vi "getEffWave.vi"(8 "error in (no error)":errorcluster, 10 "Filter Type":T1, 11 "OptStateEsti in":refnum<class "OptStateEsti.lvclass">) -> (0 "error out":errorcluster, 2 "Effective Wavelength  (um)":dbl, 3 "OptStateEsti out":refnum<class "OptStateEsti.lvclass">)   [LabVIEW 2016, in "OptStateEsti.lvclass"]
doc: "Get the effective wavelength in um based on the active filter type (u, g, r, i, z, y, ref). It is noted that \"ref\" means the monochromatic reference wavelength."
uses:
  OptStateEsti.lvclass
  StrictDef/FilterType.ctl
  OptStateEsti.lvclass/OptStateEsti.ctl
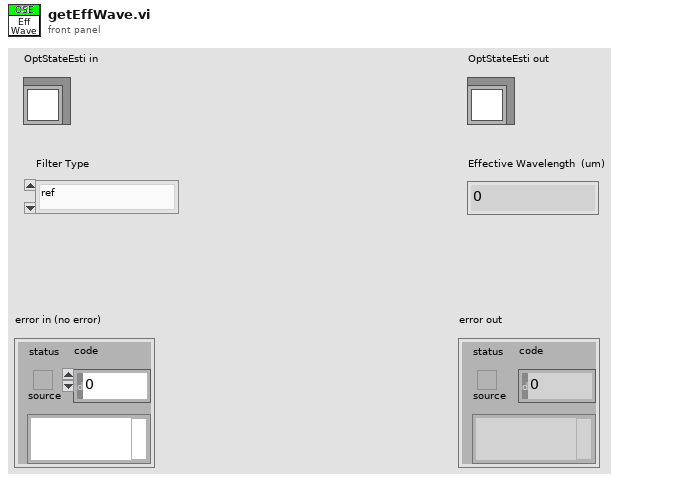
[diagram p1: front panel]
types:
  T1 = typedef "FilterType.ctl" = enum16{"ref", "u", "g", "r", "i", "z", "y"}
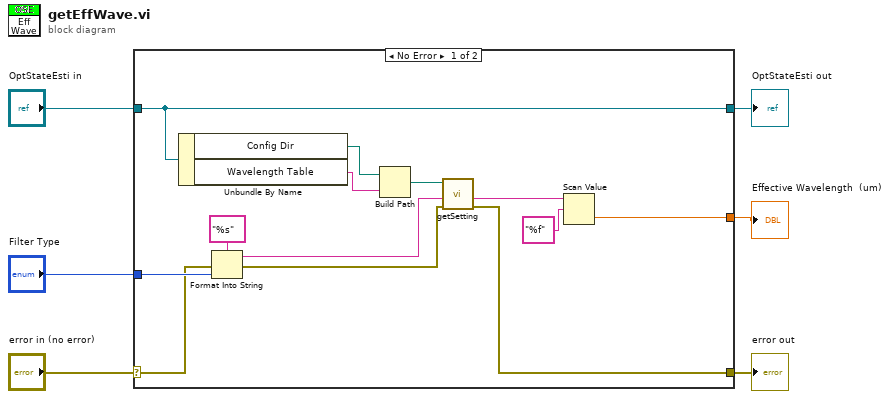
[diagram p0: block diagram]
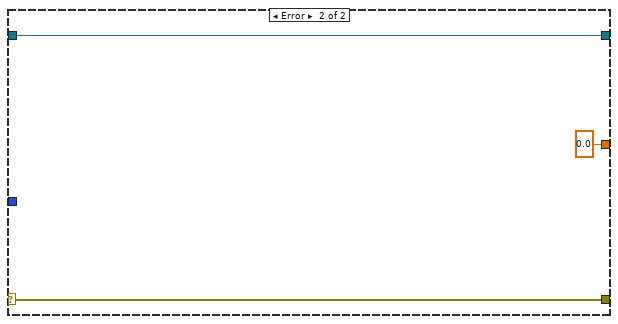
[diagram p2: hidden frame]
diagram:
  n1 = case shown="No Error" "error in (no error)" {
    selector: "error in (no error)" -> [w10 w22]
    tunnel: [w16 w22] -> w5
    tunnel: [w18 w21] -> w3
    tunnel: "OptStateEsti in" -> [w18 w21]
    tunnel: [w13 0.0] -> w2
    tunnel: "Filter Type" -> [w11 _]
    frame No Error {
      n2 = Unbundle By Name(w18) -> ("Config Dir"=w19:path, "Wavelength Table"=w7:string)
      n3 = Format Into String(format string="%s", error in=w10, w11) -> (resulting string=w9:string, error out=w8:errorcluster)  [unwired: 1 in]
      n4 = Build Path(base path=w19, name or relative path=w7) -> (appended path=w17:path)
      n5 = call "getSetting.vi"("error in"=w8, "Parameter"=w9, "Path"=w17) -> ("error out"=w16:errorcluster, "Value"=w14:string)  [unwired: 7 in]
      n6 = Scan Value(string=w14, format string="%f") -> (value=w13:dbl)  [unwired: 1 in, 1 out]
    }
    frame Error {
    }
  }
  "error out" <- w5
  "OptStateEsti out" <- w3
  "Effective Wavelength  (um)" <- w2
